vi "RatTracker - simpler UI.vi"() -> ()   [LabVIEW 2014]
panel:
  out "Image Logging Path Out":path
  out "Lost Frame Count":u32
  out "Frame Rate":dbl
  out "Raw Video":T1(plugin-control)
  in  "Stop Recording?":bool
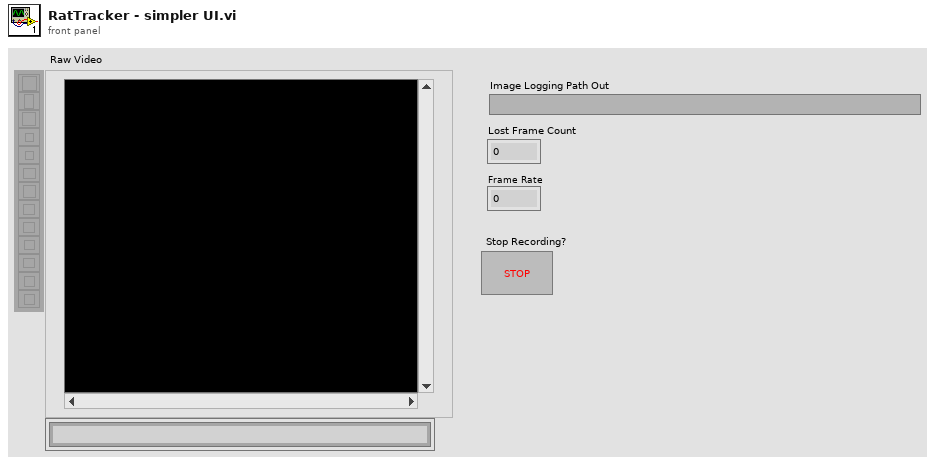
[diagram p1: front panel]
types:
  T1 = typedef "IMAQ Image.ctl" = refnum<image>
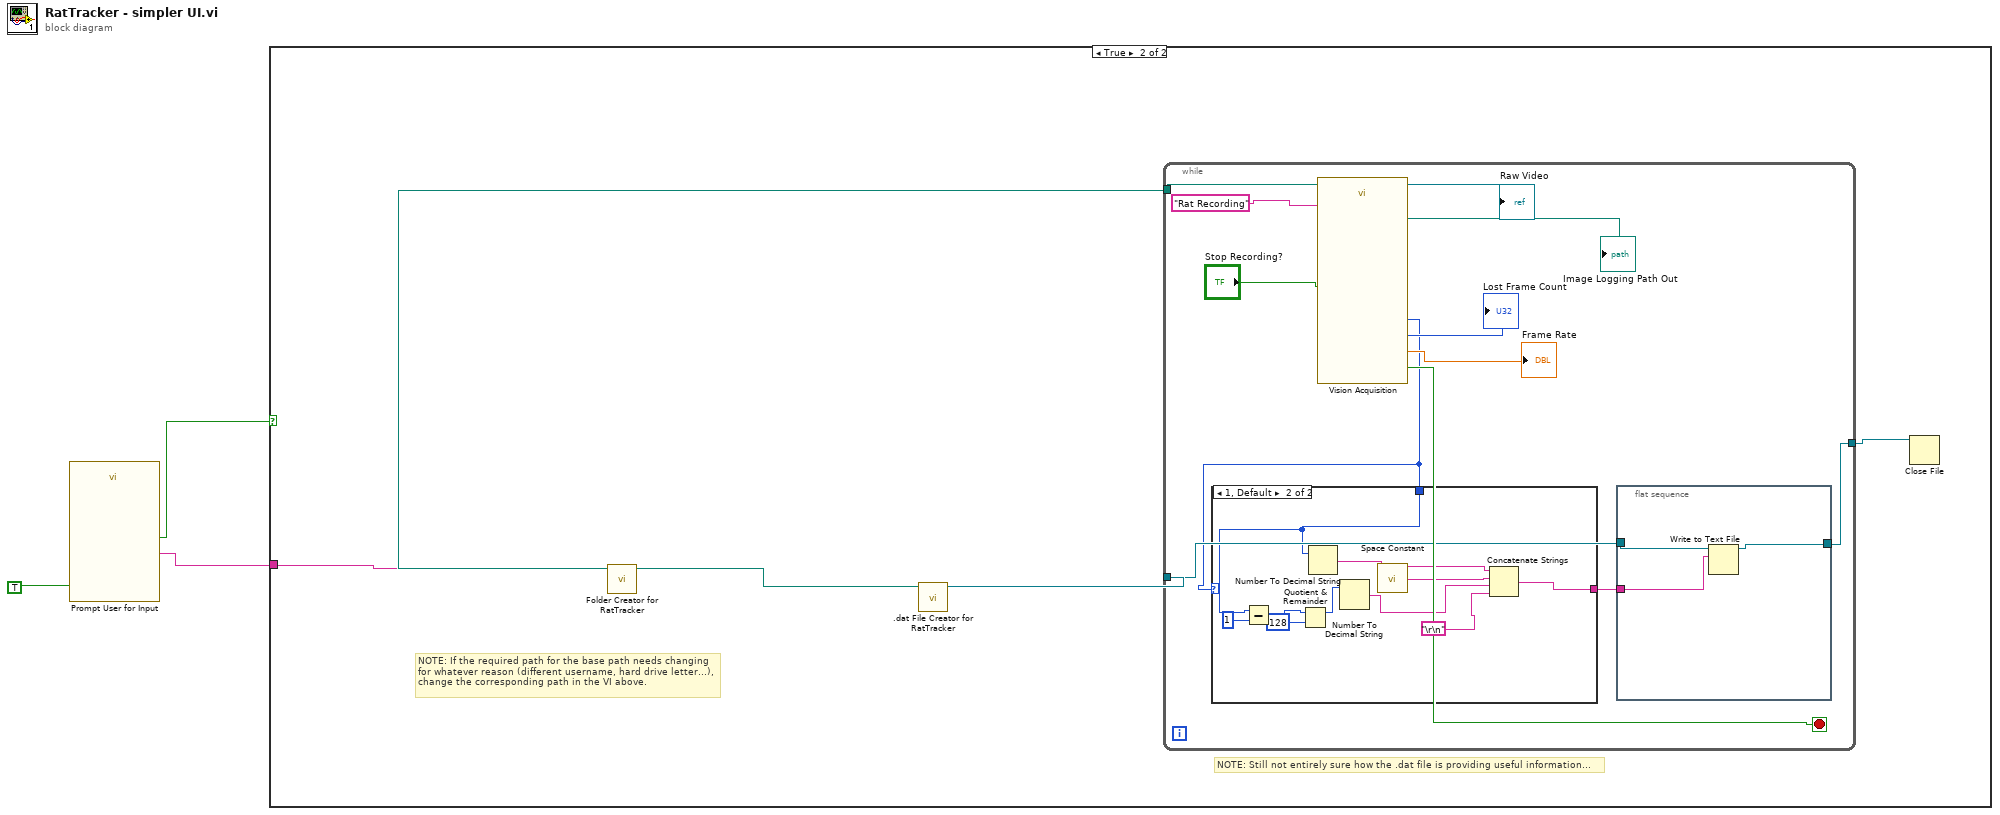
[diagram p0: block diagram]
diagram:
  n1 = call "Prompt User for Input"("Enable"=TRUE) -> ("Name"=w3:string, "OK"=w1:bool)  [unwired: 16 in, 1 out]
  n2 = case shown="True" w1 {
    tunnel: w3 -> [_ w4]
    frame False {
    }
    frame True {
      # "NOTE: If the required path for the base path needs changing\nfor whatever reason (different username, hard drive letter...),\nchange the corresponding path in the VI above."
      # "NOTE: Still not entirely sure how the .dat file is providing useful information..."
      n3 = call "Folder Creator for RatTracker.vi"("Rat Name"=w4) -> ("Path of Folder with .avi and .dat"=w5:path)  [unwired: 10 in]
      n4 = call ".dat File Creator for RatTracker.vi"("Path of Folder with .avi and .dat"=w5) -> ("Reference to .dat File"=w7:refnum<file>)  [unwired: 10 in]
      n5 = while {
        tunnel: w7 -> [w14]
        tunnel: [w12] -> w6
        tunnel: w5 -> [w10]
        stop <- w17 stop-if-true
        n6 = call "Vision Acquisition"("Image Logging Path"=w10, "Image Logging Prefix"="Rat Recording", "Stop (F)"="Stop Recording?") -> ("Image Out"=→"Raw Video":T1, "Image Number"=w11:u32, "Lost Image Count"=→"Lost Frame Count":u32, "Image Logging Path Out"=→"Image Logging Path Out":path, "Frame Rate"=→"Frame Rate":dbl, "Stopped"=w17:bool)  [unwired: 17 in, 2 out]
        n7 = case shown="1, Default" w11 {
          tunnel: [_ w27] -> w13
          tunnel: w11 -> [_ w26]
          frame 0 {
          }
          frame 1, Default {
            n8 = Subtract(x=w26, y=u32 1) -> (x-y=w24:u32)
            n9 = Quotient & Remainder(x=w24, y=u32 128) -> (x-y*floor(x/y)=w22:u32)  [unwired: 1 out]
            n10 = Number To Decimal String(number=w26) -> (decimal integer string=w28:string)  [unwired: 1 in]
            n11 = Number To Decimal String(number=w22) -> (decimal integer string=w21:string)  [unwired: 1 in]
            n12 = call <vilib>:"Space Constant.vi"() -> ("String"=w29:string)
            n13 = Concatenate Strings "Concatenate Strings"(w28, w29, w21, "\r\n") -> (w27:string)
          }
        }
        n14 = flat-sequence {
          tunnel: w14 -> [w32]
          tunnel: w13 -> [w31]
          tunnel: [w30] -> w12
          frame #0 {
            n15 = Write to Text File(file (use dialog)=w32, text=w31) -> (refnum out=w30:refnum<file>)  [unwired: 2 in, 2 out]
          }
        }
      }
      n16 = Close File(refnum=w6) -> ()  [unwired: 1 in, 2 out]
    }
  }
